vi "setChildren.vi"(8 "error in (no error)":errorcluster, 10 "Children":refnum<data-value>[](array[refnum]), 11 "TreeNode in":refnum<class "TreeNode.lvclass">) -> (0 "error out":errorcluster, 3 "TreeNode out":refnum<class "TreeNode.lvclass">)   [LabVIEW 2013, in "TreeNode.lvclass"]
doc: "Sets the children nodes."
uses:
  TreeNode.lvclass
  TreeNode.lvclass/TreeNode.ctl
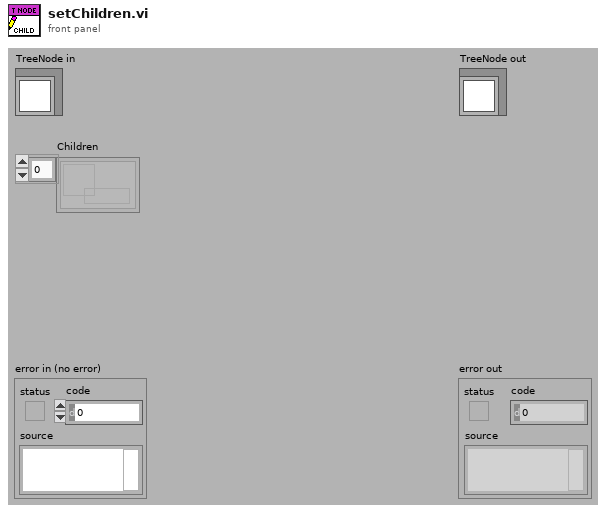
[diagram p1: front panel]
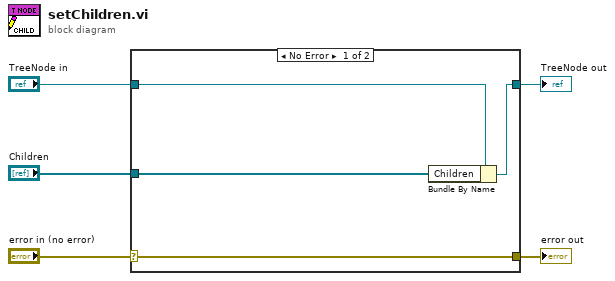
[diagram p0: block diagram]
diagram:
  n1 = case shown="No Error" "error in (no error)" {
    selector: "error in (no error)" -> [w9 w10]
    tunnel: [w9 w10] -> w4
    tunnel: [w7 w11] -> w2
    tunnel: "TreeNode in" -> [w8 w11]
    tunnel: "Children" -> [w6 _]
    frame No Error {
      n2 = Bundle By Name(cluster=w8, "Children"=w6) -> (w7:refnum<class "TreeNode.lvclass">)
    }
    frame Error {
    }
  }
  "error out" <- w4
  "TreeNode out" <- w2
